vi "Read selection.vi"(8 "error in (no error)":errorcluster, 11 "Cursor in":refnum<class "Cursor.lvclass">) -> (0 "error out":errorcluster, 2 "selection":i16, 3 "Cursor out":refnum<class "Cursor.lvclass">)   [LabVIEW 2019, in "RT_Game.lvlib" / "Cursor.lvclass"]
uses:
  Cursor.lvclass
  Cursor.lvclass/Cursor.ctl
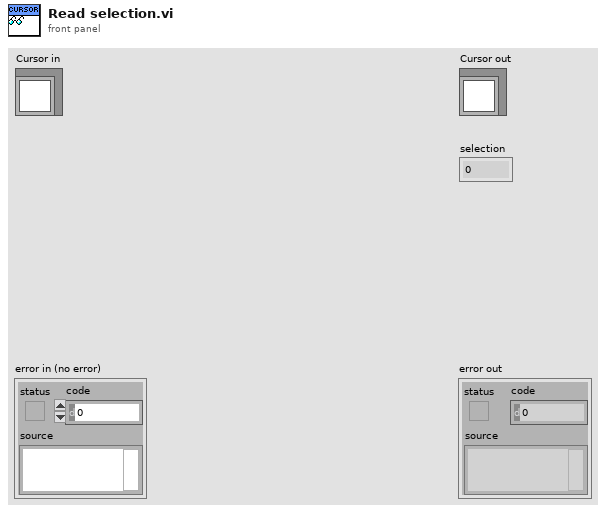
[diagram p1: front panel]
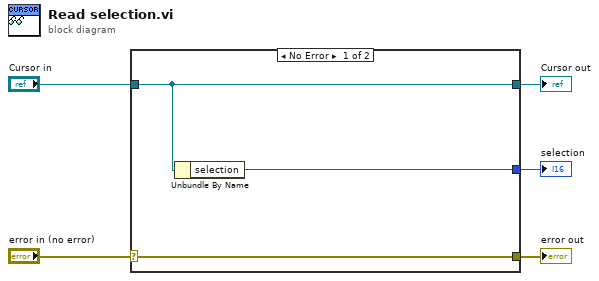
[diagram p0: block diagram]
diagram:
  n1 = case shown="No Error" "error in (no error)" {
    selector: "error in (no error)" -> [w8 w9]
    tunnel: [w8 w9] -> w4
    tunnel: [w7 w10] -> w2
    tunnel: "Cursor in" -> [w7 w10]
    tunnel: [w6 _] -> w1
    frame No Error {
      n2 = Unbundle By Name(w7) -> ("selection"=w6:i16)
    }
    frame Error {
    }
  }
  "error out" <- w4
  "Cursor out" <- w2
  "selection" <- w1
